vi "PidFunc.vi"(6 "刹车":bool, 11 "运用学解算后得\n到的两个电机\n的期望角速度":dbl[](array[numeric])=[0.0] caption="设定值" format="%.2f") -> (3 "得到电机转动的角速度":dbl[](array[numeric]))   [LabVIEW 2017]
uses:
  <vilib>/myRIO/Common/Instrument Driver Framework/myRIO v1.0/Encoder/typedefs/Encoder Signal Mode.ctl
  <vilib>/myRIO/Instrument Drivers/Onboard IO/Encoder/typedefs/Encoder Reference.ctl
  <vilib>/myRIO/Common/Instrument Driver Framework/Utilities/typedefs/myRIO Generic Hardware Reference.ctl
  <vilib>/myRIO/Common/Instrument Driver Framework/Utilities/typedefs/Hardware Version Enum.ctl
  <vilib>/myRIO/Common/Instrument Driver Framework/Utilities/typedefs/myRIO v1.0 Reference.ctl
  <vilib>/myRIO/Common/Instrument Driver Framework/Utilities/typedefs/Generic FPGA Reference.ctl
  <vilib>/myRIO/Common/Instrument Driver Framework/myRIO v1.0/Encoder/typedefs/Encoder Channels Enum.ctl
  <vilib>/myRIO/Common/Instrument Driver Framework/myRIO v1.0/Encoder/typedefs/Encoder Configuration v1.0.ctl
  <vilib>/userdefined/High Color/nirio_resource_hc.ctl
  <vilib>/myRIO/Instrument Drivers/Onboard IO/DIO/typedefs/DIO Reference.ctl
  <vilib>/myRIO/Common/Instrument Driver Framework/myRIO v1.0/DIO/typedefs/DIO Channels List.ctl
  <vilib>/myRIO/Common/Instrument Driver Framework/myRIO v1.0/DIO/typedefs/DIO Channels Enum.ctl
  <vilib>/myRIO/Instrument Drivers/Onboard IO/PWM/typedefs/PWM Reference.ctl
  <vilib>/myRIO/Common/Instrument Driver Framework/myRIO v1.0/PWM/typedefs/PWM Channels Enum.ctl
  <vilib>/myRIO/Instrument Drivers/Onboard IO/PWM/typedefs/PWM Configuration.ctl
  <vilib>/myRIO/Common/Instrument Driver Framework/Utilities/vis/Is FPGA Ref Available.vi
  <vilib>/myRIO/Common/Instrument Driver Framework/myRIO v1.0/Encoder/vis/myRIO v1.1 Open Encoder.vi
  <vilib>/myRIO/Instrument Drivers/Onboard IO/Encoder/vis/Read.vi
  <vilib>/myRIO/Common/Instrument Driver Framework/myRIO v1.0/DIO/vis/myRIO v1.1 Open DIO.vi
  <vilib>/myRIO/Instrument Drivers/Onboard IO/DIO/vis/Write.vi
  <vilib>/myRIO/Common/Instrument Driver Framework/myRIO v1.0/PWM/vis/myRIO v1.1 Open PWM.vi
  <vilib>/myRIO/Instrument Drivers/Onboard IO/PWM/vis/Set Duty Cycle and Frequency.vi
  <vilib>/myRIO/Common/Instrument Driver Framework/Utilities/vis/Validate Channels.vi
  <vilib>/myRIO/Common/Instrument Driver Framework/myRIO v1.0/Encoder/vis/myRIO v1.0 Reserve Encoder.vi
  <vilib>/myRIO/Common/Instrument Driver Framework/myRIO v1.0/DIO/vis/myRIO v1.0 Reserve DIO.vi
  <vilib>/myRIO/Common/Instrument Driver Framework/myRIO v1.0/PWM/vis/myRIO v1.0 Reserve PWM.vi
  <vilib>/myRIO/Common/Instrument Driver Framework/myRIO v1.0/Encoder/vis/myRIO v1.0 Build MUX Configuration Encoder.vi
  <vilib>/myRIO/Common/Instrument Driver Framework/myRIO v1.0/Resource Manager/vis/myRIO v1.0 Reserve Channel List.vi
  <vilib>/myRIO/Common/Instrument Driver Framework/myRIO v1.0/DIO/vis/myRIO v1.0 Build MUX Configuration DIO.vi
  <vilib>/myRIO/Common/Instrument Driver Framework/myRIO v1.0/PWM/vis/myRIO v1.0 Build MUX Configuration PWM.vi
  <vilib>/myRIO/Common/Instrument Driver Framework/myRIO v1.0/Resource Manager/vis/myRIO v1.0 Create Configuration List.vi
  <vilib>/myRIO/Common/Instrument Driver Framework/myRIO v1.0/Resource Manager/vis/myRIO v1.0 Reserve Channel.vi
  <vilib>/myRIO/Common/Instrument Driver Framework/myRIO v1.0/Resource Manager/vis/myRIO v1.0 Unreserve Channel.vi
  <vilib>/myRIO/Common/Instrument Driver Framework/myRIO v1.0/Resource Manager/vis/myRIO v1.0 Build Mutex Name.vi
  <vilib>/Utility/VariantDataType/GetNumericInfo.vi
  <vilib>/Utility/error.llb/Error Cluster From Error Code.vi
  <vilib>/myRIO/Common/Instrument Driver Framework/myRIO v1.0/myRIO v1.1 Open.vi
  <vilib>/myRIO/Common/Instrument Driver Framework/Utilities/vis/IO Manager.vi
  <vilib>/myRIO/Common/Instrument Driver Framework/Utilities/vis/Configuration Manager.vi
  <vilib>/myRIO/Common/Instrument Driver Framework/myRIO v1.0/Resource Manager/vis/myRIO v1.0 Configure IO.vi
  <vilib>/myRIO/Common/Instrument Driver Framework/myRIO v1.0/myRIO v1.0 Close.vi
  <vilib>/myRIO/Common/Instrument Driver Framework/myRIO v1.0/Encoder/vis/myRIO v1.0 Configure Encoder.vi
  <vilib>/myRIO/Common/Instrument Driver Framework/myRIO v1.0/Encoder/vis/myRIO v1.0 Read Encoder.vi
  <vilib>/addons/control/pid/pid.llb/PID (DBL Array).vi
  <vilib>/myRIO/Common/Instrument Driver Framework/myRIO v1.0/DIO/vis/myRIO v1.0 Write DIO.vi
  <vilib>/myRIO/Common/Instrument Driver Framework/myRIO v1.0/PWM/vis/myRIO v1.0 Write PWM.vi
  <vilib>/myRIO/Express VI/Onboard IO/Encoder/Encoder Express VI.xnode
  <vilib>/myRIO/Instrument Drivers/Onboard IO/Encoder/vis/myRIO Encoder Open.xnode
  <vilib>/myRIO/Common/Instrument Driver Framework/myRIO v1.0/Encoder/typedefs/Encoder Count Direction Enum.ctl
  <vilib>/myRIO/Express VI/Onboard IO/DO/DO Express VI.xnode
  <vilib>/myRIO/Instrument Drivers/Onboard IO/DIO/vis/myRIO DIO Open.xnode
  <vilib>/myRIO/Express VI/Onboard IO/PWM/PWM Express VI.xnode
  <vilib>/myRIO/Instrument Drivers/Onboard IO/PWM/vis/myRIO PWM Open.xnode
  <vilib>/myRIO/Instrument Drivers/Onboard IO/Encoder/Encoder.lvlib
  <vilib>/addons/control/pid/NI_PID_pid.lvlib
  <vilib>/myRIO/Instrument Drivers/Onboard IO/PWM/PWM.lvlib
  <vilib>/myRIO/Instrument Drivers/Onboard IO/DIO/DIO.lvlib
panel:
  out "编码器差值\n0->右编码器\n1->左编码器":i32[](array[numeric])
  out "编码器数值\n0->右编码器\n1->左编码器":i32[](array[numeric])
  out "波形图表":cluster{"setpoint":dbl, "Counter Value":dbl}(graph)
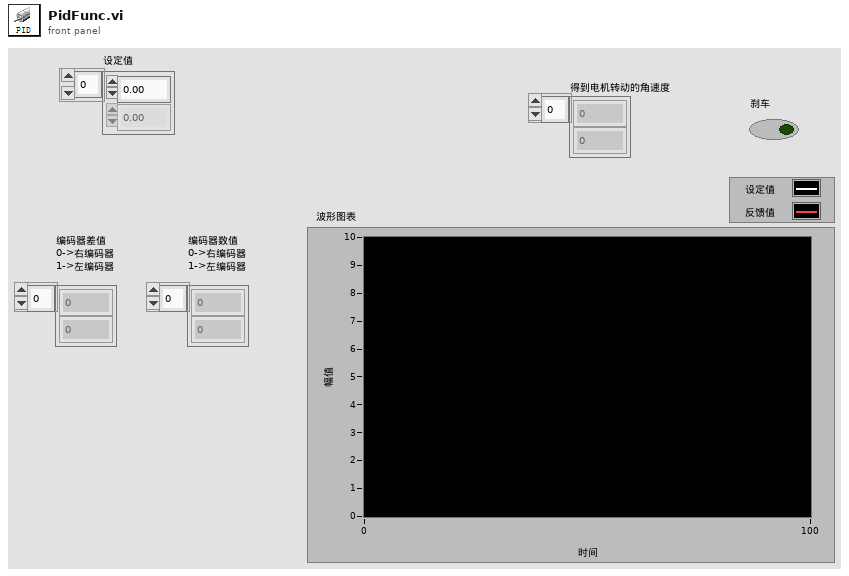
[diagram p1: front panel]
types:
  T1 = cluster{"proportional gain (Kc)":dbl, "integral time (Ti, min)":dbl, "derivative time (Td, min)":dbl}[]
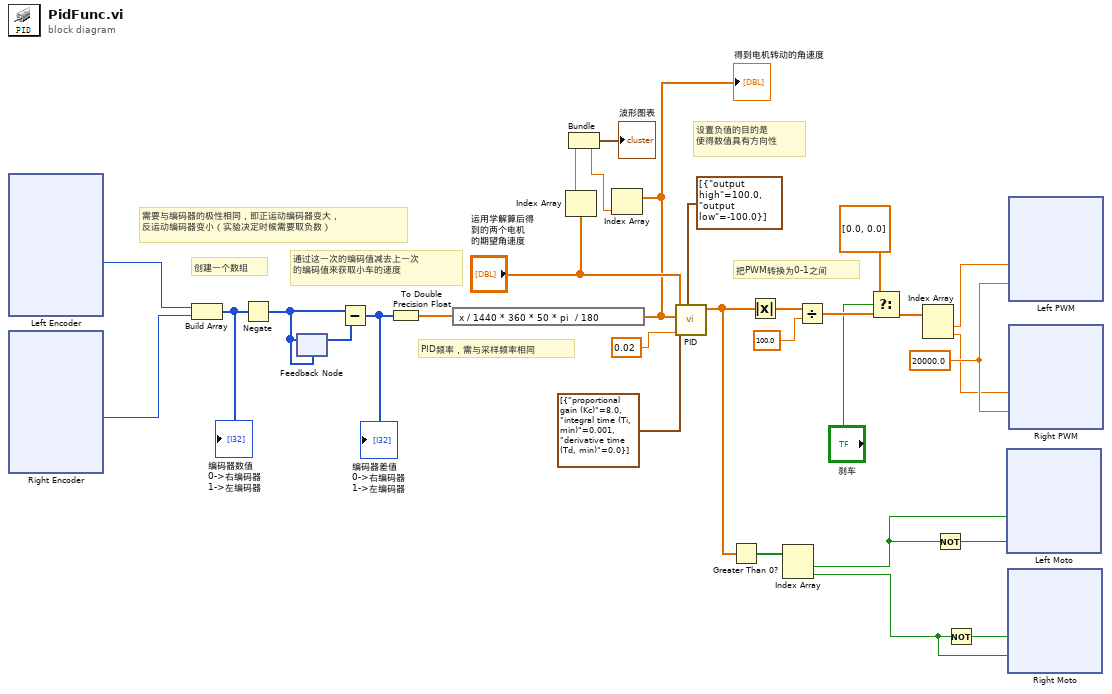
[diagram p0: block diagram]
diagram:
  w24 = 20000.0 ("Frequency [Hz]")
  # "设置负值的目的是\n使得数值具有方向性"
  # "PID频率，需与采样频率相同"
  # "把PWM转换为0-1之间"
  # "通过这一次的编码值减去上一次\n的编码值来获取小车的速度"
  # "需要与编码器的极性相同，即正运动编码器变大，\n反运动编码器变小（实验决定时候需要取负数）"
  # "创建一个数组"
  n1 = xnode "Left Encoder"() -> ("Counter Value"=w6:i32)  [unwired: 2 in, 3 out]
  n2 = xnode "Right Encoder"() -> ("Counter Value"=w5:i32)  [unwired: 2 in, 3 out]
  n3 = Build Array(w6, w5) -> (w23:i32[])
  "编码器数值\n0->右编码器\n1->左编码器" <- w23
  n4 = Negate(x=w23) -> (-x=w30:i32[])
  n5 = feedback #1(w30) -> (w29:i32[])
  n6 = feedback-in #1(w30) -> ()
  n7 = Subtract(x=w30, y=w29) -> (x-y=w22:i32[])
  "编码器差值\n0->右编码器\n1->左编码器" <- w22
  n8 = To Double Precision Float(number=w22) -> (double precision float=w28:dbl[])
  n9 = expression code="x / 1440 * 360 * 50 * pi  / 180"(w28) -> (w18:dbl[])
  "得到电机转动的角速度" <- w18
  n10 = Index Array(array="运用学解算后得\n到的两个电机\n的期望角速度") -> (element=w17:dbl)  [unwired: 1 in]
  n11 = Index Array(array=w18) -> (element=w16:dbl)  [unwired: 1 in]
  n12 = Bundle("setpoint"=w17, "Counter Value"=w16) -> (→"波形图表":cluster{"setpoint":dbl, "Counter Value":dbl})  [unwired: 1 in]
  n13 = call-poly <vilib>:"PID.vi"("output range"=cluster{"output high":dbl, "output low":dbl}[] [{"output high"=100.0, "output low"=-100.0}], "dt (s)"=0.02, "PID gains"=T1 [{"proportional gain (Kc)"=8.0, "integral time (Ti, min)"=0.001, "derivative time (Td, min)"=0.0}], "process variable"=w18, "setpoint"="运用学解算后得\n到的两个电机\n的期望角速度") -> ("output"=w21:dbl[])  [unwired: 5 in, 1 out]
  n14 = Greater Than 0?(x=w21) -> (x > 0?=w20:bool[])
  n15 = Absolute Value(x=w21) -> (abs(x)=w26:dbl[])
  n16 = Index Array(array=w20) -> (element #1=w2:bool, element #2=w1:bool)  [unwired: 2 in]
  n17 = Divide(x=w26, y=100.0) -> (x/y=w14:dbl[])
  n18 = Select(t=dbl[] [0.0, 0.0], s="刹车", f=w14) -> (s? t:f=w13:dbl[])
  n19 = Index Array(array=w13) -> (element #1=w4:dbl, element #2=w3:dbl)  [unwired: 2 in]
  n20 = Not(x=w2) -> (.not. x?=w8:bool)
  n21 = Not(x=w1) -> (.not. x?=w9:bool)
  n22 = xnode "Left Moto"("A/DIO7 (Pin 25)"=w2, "A/DIO13 (Pin 26)"=w8) -> ()  [unwired: 1 in, 1 out]
  n23 = xnode "Right Moto"("A/DIO5 (Pin 21)"=w9, "A/DIO6 (Pin 23)"=w1) -> ()  [unwired: 1 in, 1 out]
  n24 = xnode "Left PWM"("Duty Cycle"=w4, "Frequency [Hz]"=w24) -> ()  [unwired: 1 in, 1 out]
  n25 = xnode "Right PWM"("Duty Cycle"=w3, "Frequency [Hz]"=w24) -> ()  [unwired: 1 in, 1 out]
